vi "Write Steps.vi"(8 "error in (no error)":errorcluster, 10 "Steps":refnum<class "Step Config.lvclass">[](array[class]), 11 "StepCategoryNode in":refnum<class "CleanupCategoryNode.lvclass">) -> (0 "error out":errorcluster, 3 "StepCategoryNode out":refnum<class "CleanupCategoryNode.lvclass">)   [LabVIEW 2015, in "CleanupCategoryNode.lvclass"]
uses:
  CleanupCategoryNode.lvclass
  Prototype/classes/Step/Config/Step Config.lvclass
  CleanupCategoryNode.lvclass/CleanupCategoryNode.ctl
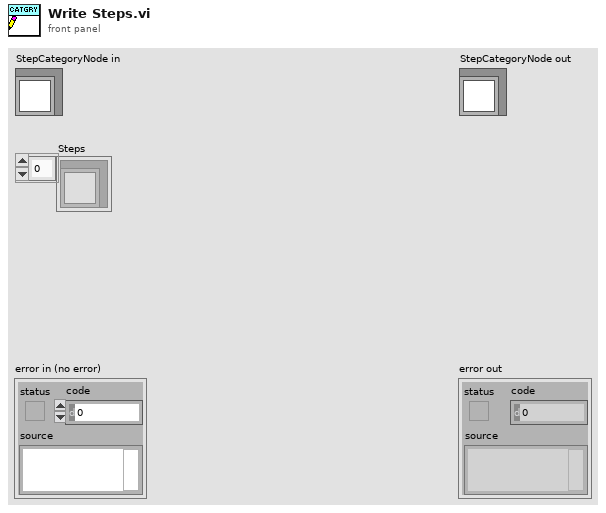
[diagram p1: front panel]
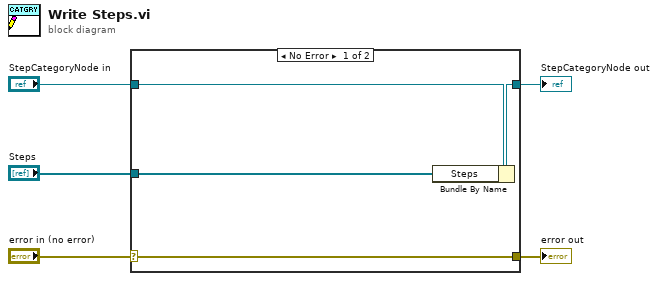
[diagram p0: block diagram]
diagram:
  n1 = case shown="No Error" "error in (no error)" {
    selector: "error in (no error)" -> [w9 w10]
    tunnel: [w9 w10] -> w4
    tunnel: [w7 w11] -> w2
    tunnel: "StepCategoryNode in" -> [w8 w11]
    tunnel: "Steps" -> [w6 _]
    frame No Error {
      n2 = Bundle By Name(cluster=w8, "Steps"=w6) -> (w7:refnum<class "CleanupCategoryNode.lvclass">)
    }
    frame Error {
    }
  }
  "error out" <- w4
  "StepCategoryNode out" <- w2
